vi "Update Pin Map.vi"(0 "Pin Map Path":string, 2 "Sequence Context In":refnum<k7>, 3 "error in":errorcluster) -> (10 "error out":errorcluster)   [LabVIEW 2020, in "NIDigitalBurstPattern.lvlib"]
uses:
  NIDigitalBurstPattern.lvlib
  <vilib>/MeasurementLink/MeasurementLink Measurement Server/MeasurementLink Measurement Server.lvlib
  <vilib>/MeasurementLink/MeasurementLink Discovery Client/MeasurementLink Discovery Client.lvlib
  <vilib>/MeasurementLink/MeasurementLink Discovery Client/RPC Messages/ni_measurementlink_discovery_v1_ResolveServiceRequest.ctl
  <vilib>/MeasurementLink/MeasurementLink Pin Map Client/MeasurementLink Pin Map Client.lvlib
  <vilib>/MeasurementLink/MeasurementLink Pin Map Client/RPC Messages/ni_measurementlink_pinmap_v1_UpdatePinMapFromXmlRequest.ctl
  Measurement Service Helpers/Measurement Service Helpers.lvlib
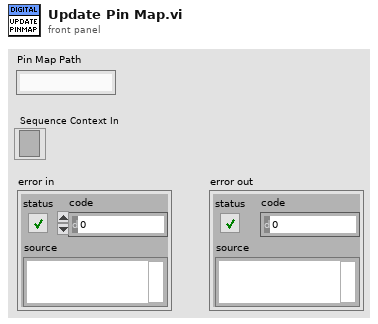
[diagram p1: front panel]
types:
  T1 = typedef "MeasurementLink Pin Map Client.lvlib/ni_measurementlink_pinmap_v1_UpdatePinMapFromXmlRequest.ctl" = cluster{"pin_map_id":string, "pin_map_xml":string}
  T2 = typedef "MeasurementLink Discovery Client.lvlib/ni_measurementlink_discovery_v1_ResolveServiceRequest.ctl" = cluster{"provided_interface":string, "service_class":string}
  T3 = typedef "grpc-lvsupport-release.lvlib/grpcId.ctl" = u64
  T4 = typedef "MeasurementLink Discovery Client.lvlib/ni_measurementlink_discovery_v1_ServiceLocation.ctl" = cluster{"location":string, "insecure_port":string, "ssl_authenticated_port":string}
  T5 = typedef "MeasurementLink Pin Map Client.lvlib/ni_measurementlink_pinmap_v1_PinMap.ctl" = cluster{"pin_map_id":string}
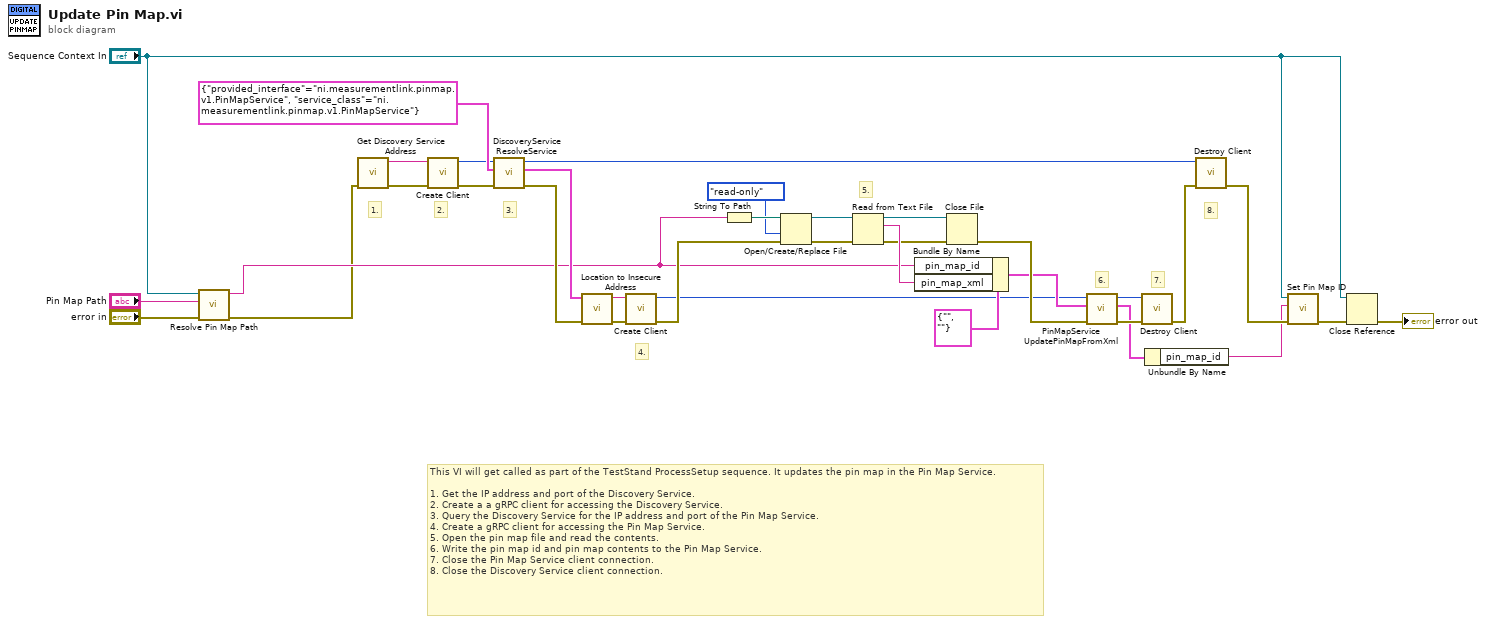
[diagram p0: block diagram]
diagram:
  # "8."
  # "7."
  # "6."
  # "5."
  # "4."
  # "3."
  # "2."
  # "1."
  # "This VI will get called as part of the TestStand ProcessSetup sequence. It updates the pin map in the Pin Map Service. \n\n1. Get the IP address and port of the Discovery Service.\n2. Create a a gRPC client for accessing the Discovery Service.\n3. Query the Discovery Service for the IP address and port of the Pin Map Service.\n4. Create a gRPC client for accessing the Pin Map Service.\n5. Open the pin map file and read the contents.\n6. Write the pin map id and pin map contents to the Pin Map Service.\n7. Close the Pin Map Service client connection.\n8. Close the Discovery Service client connection."
  n1 = call "Resolve Pin Map Path.vi"("error in"="error in", "Pin Map Path"="Pin Map Path", "Sequence Context In"="Sequence Context In") -> ("error out"=w8:errorcluster, "Pin Map Path"=w9:string)  [unwired: 7 in]
  n2 = call <vilib>:"Get Discovery Service Address.vi"("error in"=w8) -> ("error out"=w34:errorcluster, "address"=w33:string)  [unwired: 9 in]
  n3 = call <vilib>:"Create Client.vi"("error in"=w34, "address"=w33) -> ("error out"=w23:errorcluster, "gRPC ID Out"=w31:T3)  [unwired: 8 in]
  n4 = call <vilib>:"DiscoveryService ResolveService.vi"("error in"=w23, "Request Data"=T2 {"provided_interface"="ni.measurementlink.pinmap.v1.PinMapService", "service_class"="ni.measurementlink.pinmap.v1.PinMapService"}, "gRPC ID"=w31) -> ("error out"=w22:errorcluster, "Response Data"=w12:T4, "gRPC ID out"=w13:T3)  [unwired: 6 in]
  n5 = call "Location to Insecure Address.vi"("Location"=w12) -> ("String"=w11:string)  [unwired: 10 in]
  n6 = call <vilib>:"Create Client.vi"("error in"=w22, "address"=w11) -> ("error out"=w21:errorcluster, "gRPC ID Out"=w17:T3)  [unwired: 8 in]
  n7 = String To Path(string=w9) -> (path=w30:path)
  n8 = Open/Create/Replace File(file path (use dialog)=w30, error in=w21, access (0:read/write)=enum16{"read/write", "read-only", "write-only"}."read-only") -> (refnum out=w27:refnum<file>, error out=w28:errorcluster)  [unwired: 3 in, 1 out]
  n9 = Read from Text File(file (use dialog)=w27, error in=w28) -> (refnum out=w24:refnum<file>, text=w26:string, error out=w25:errorcluster)  [unwired: 2 in, 1 out]
  n10 = Bundle By Name(cluster=T1 {"pin_map_id"="", "pin_map_xml"=""} ("Request Data"), "pin_map_id"=w9, "pin_map_xml"=w26) -> (w18:T1)
  n11 = Close File(refnum=w24, error in=w25) -> (error out=w20:errorcluster)  [unwired: 1 out]
  n12 = call <vilib>:"PinMapService UpdatePinMapFromXml.vi"("error in"=w20, "Request Data"=w18, "gRPC ID"=w17) -> ("error out"=w16:errorcluster, "Response Data"=w10:T5, "gRPC ID out"=w15:T3)  [unwired: 6 in]
  n13 = call <vilib>:"Destroy Client.vi"("error in"=w16, "gRPC ID"=w15) -> ("error out"=w14:errorcluster)  [unwired: 9 in]
  n14 = Unbundle By Name(w10) -> ("pin_map_id"=w2:string)
  n15 = call <vilib>:"Destroy Client.vi"("error in"=w14, "gRPC ID"=w13) -> ("error out"=w7:errorcluster)  [unwired: 9 in]
  n16 = call "Set Pin Map ID.vi"("error in"=w7, "pin_map_id"=w2, "Sequence Context"="Sequence Context In") -> ("error out"=w6:errorcluster)  [unwired: 8 in]
  n17 = Close Reference(reference="Sequence Context In", error in (no error)=w6) -> (error out=→"error out":errorcluster)
